vi "writeBuffer.vi"(0 "dataSize":i32, 1 "meta":T1={"DYB_Order"=2, "Spalte"=2, "Zeile"=260, "Abstand Datenpunkte"=5.757235038420917e+29, "Abstand Scanzeilen"=-5.4779473692595377e+23, "x-Koordinate 1. Punkt"=3.18299368645e-313, "y-Koordinate 2. Punkt"=0.007812501473381417, "Neigungswinkel Scanfeld"=8.487983164e-314, "Einheit Variablen"=2, "stepVal"=0.0, "stepValNum"=0.0, "offsetVal"=0.0, "unitVal"=2}, 2 "index":i32, 4 "data":i32[](array[numeric]), 5 "error in":T3, 6 "comment":string, 7 "binary":bool=TRUE, 8 "fileName":string, 9 "forward":bool=TRUE) -> (19 "error out":T2)   [LabVIEW 2016]
doc: "Writes the data from the \"data\"-array into a file. We recommend to use the VI 'writeMultiBuffer.vi' instead of this one. The inputs are:\n- fileName: Name of the file to be created. You can also pass a whole path to that input. Note that you have to escape the slash(es) in the path.\n- Comment: String that will be written into the header of the generated file\n- DataSize: Number of data points (32-bit elements) to be written to a file\n- Meta: Meta data for the buffer as retrieved by getDataBuffer\n- Index: index of first element in the buffer\n- Data: data buffer as retrieved by getDataBuffer\n- Binary: True if binary format is required. Only for scan-triggered data\n- Forward: If only the data from the forward scan is to be written. Only relevant for scan-triggered data."
uses:
  Controls/Error_In.ctl
  Controls/Error_Out.ctl
  Controls/Metadata-Cluster.ctl
  Files_ASC500/DLL/daisybase.dll
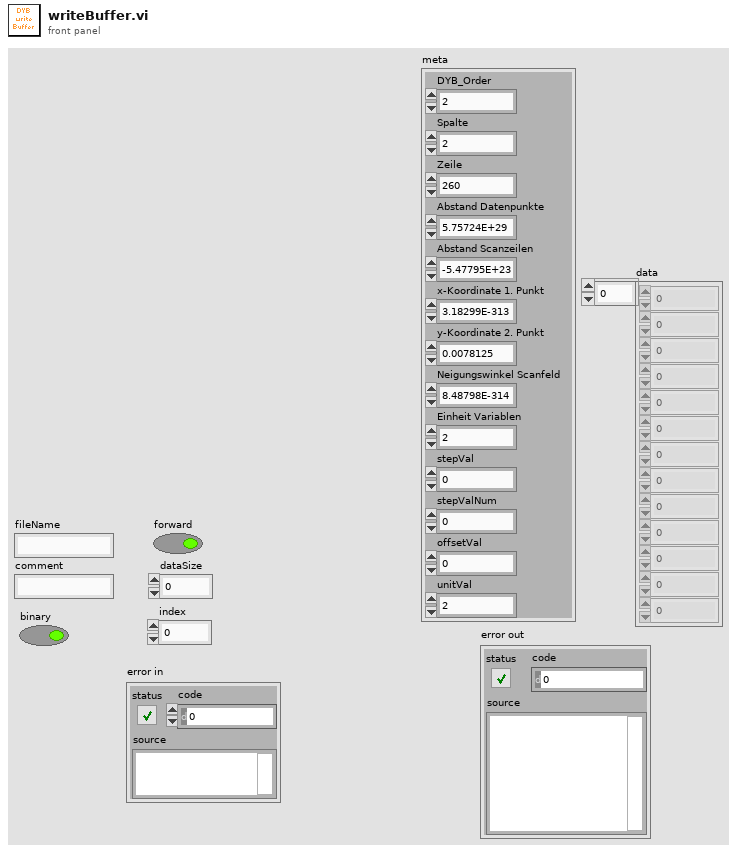
[diagram p1: front panel]
types:
  T1 = typedef "Metadata-Cluster.ctl" = cluster{"DYB_Order":i32, "Spalte":i32, "Zeile":i32, "Abstand Datenpunkte":dbl, "Abstand Scanzeilen":dbl, "x-Koordinate 1. Punkt":dbl, "y-Koordinate 2. Punkt":dbl, "Neigungswinkel Scanfeld":dbl, "Einheit Variablen":i32, "stepVal":dbl, "stepValNum":dbl, "offsetVal":dbl, "unitVal":i32}
  T2 = typedef "Error_Out.ctl" = errorcluster
  T3 = typedef "Error_In.ctl" = errorcluster
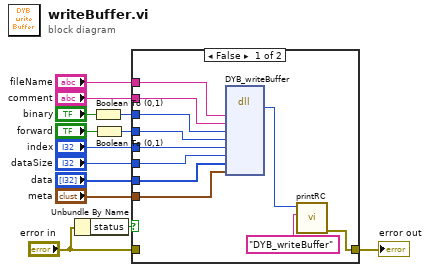
[diagram p0: block diagram]
diagram:
  n1 = Unbundle By Name("error in") -> ("status"=w13:bool)
  n2 = Boolean To (0,1)(Boolean="binary") -> (0, 1=w7:i16)
  n3 = Boolean To (0,1)(Boolean="forward") -> (0, 1=w6:i16)
  n4 = case shown="False" w13 {
    tunnel: "error in" -> [_ w25]
    tunnel: [w22 w25] -> w11
    tunnel: "dataSize" -> [w21 _]
    tunnel: w7 -> [w20 _]
    tunnel: w6 -> [w19 _]
    tunnel: "comment" -> [w18 _]
    tunnel: "fileName" -> [w17 _]
    tunnel: "index" -> [w16 _]
    tunnel: "data" -> [w15 _]
    tunnel: "meta" -> [w14 _]
    frame False {
      n5 = dll-call lib="G:/SCMOperations/Share/ELE/Produkt Information/ASC500/04 Remote Control/02 development versions/2018Nov06/Files_ASC500/DLL/daisybase.dll" fn="DYB_writeBuffer"("fileName"=w17, "comment"=w18, "binary"=w20, "forward"=w19, "index"=w16, "dataSize"=w21, "data"=w15, "meta"=w14) -> ("RC"=w24:i32)  [unwired: 11 in, 2 out]
      n6 = call "printRC.vi"("additional information"="DYB_writeBuffer", "RC"=w24) -> ("error out"=w22:T2)  [unwired: 9 in]
    }
    frame True {
    }
  }
  "error out" <- w11
